vi "HeatFlow HW Conf Save.vi"(8 "HeatFlow HW Cfg":T1, 10 "Conf File":path) -> (0 "error out":errorcluster)   [LabVIEW 2019, in "Acquisition.lvlib"]
uses:
  Acquisition.lvlib
  HeatFlow HW Cfg.ctl
  HeatFlow Acq States.ctl
  <vilib>/Utility/config.llb/Write Key (Boolean).vi
  <vilib>/Utility/config.llb/Write Key (Double).vi
  <vilib>/Utility/config.llb/Write Key (String).vi
  <vilib>/Utility/config.llb/NI_LVConfig.lvlib
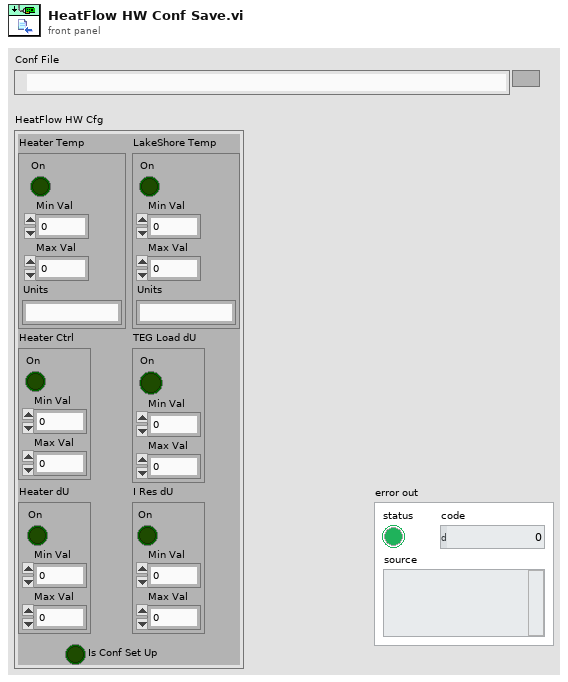
[diagram p1: front panel]
types:
  T1 = typedef "Acquisition.lvlib/HeatFlow HW Cfg.ctl" = cluster{"Heater Temp":cluster{"On":bool, "Min Val":dbl, "Max Val":dbl, "Units":string}, "LakeShore Temp":cluster{"On":bool, "Min Val":dbl, "Max Val":dbl, "Units":string}, "Heater Ctrl":cluster{"On":bool, "Min Val":dbl, "Max Val":dbl}, "TEG Load dU":cluster{"On":bool, "Min Val":dbl, "Max Val":dbl}, "Heater dU":cluster{"On":bool, "Min Val":dbl, "Max Val":dbl}, "I Res dU":cluster{"On":bool, "Min Val":dbl, "Max Val":dbl}, "Is Conf Set Up":bool}
  T2 = typedef "Acquisition.lvlib/HeatFlow Acq States.ctl" = enum16{"Start", "--- Control ---", "HeaterTemp", "DoControl?", "HeaterCtrl", "--- Readings ---", "DoReadings?", "I_Res_dU", "LakeShoreTemp", "Heater_dU", "TEG_Load_dU", "Calculations", "End"}
  T3 = typedef "NI_LVConfig.lvlib/Config Data RefNum.ctl" = refnum<k1>
  T4 = cluster{"On":bool, "Min Val":dbl, "Max Val":dbl, "Units":string}
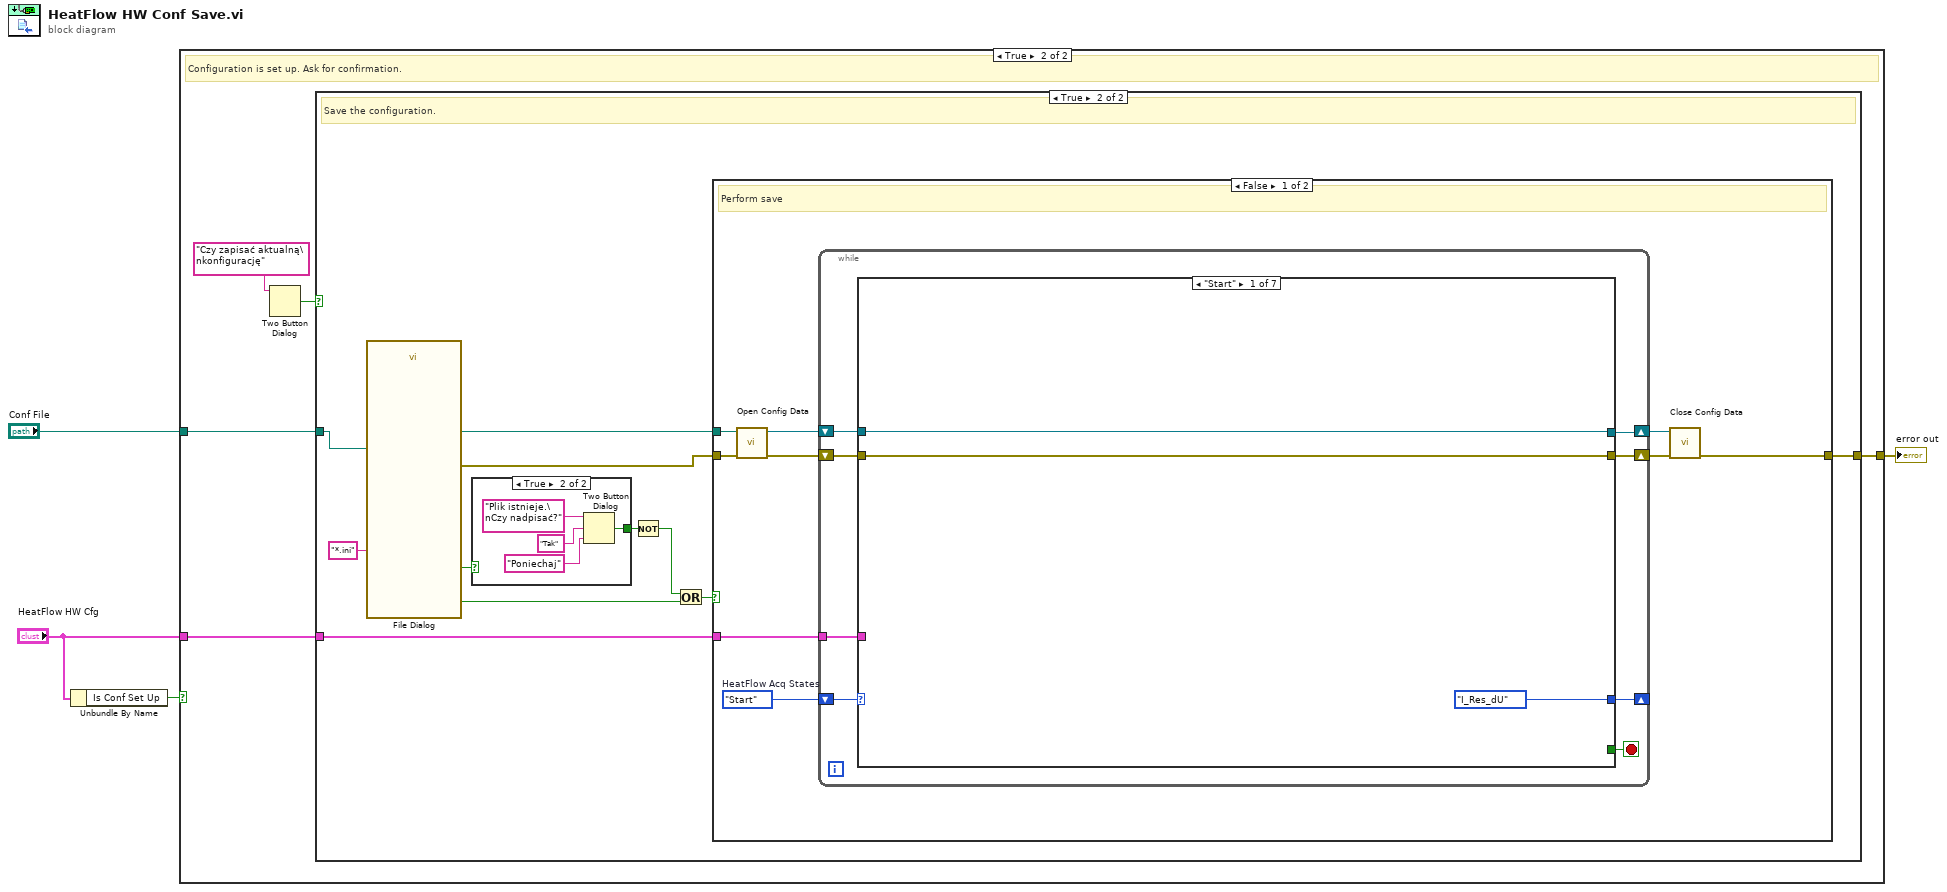
[diagram p0: block diagram]
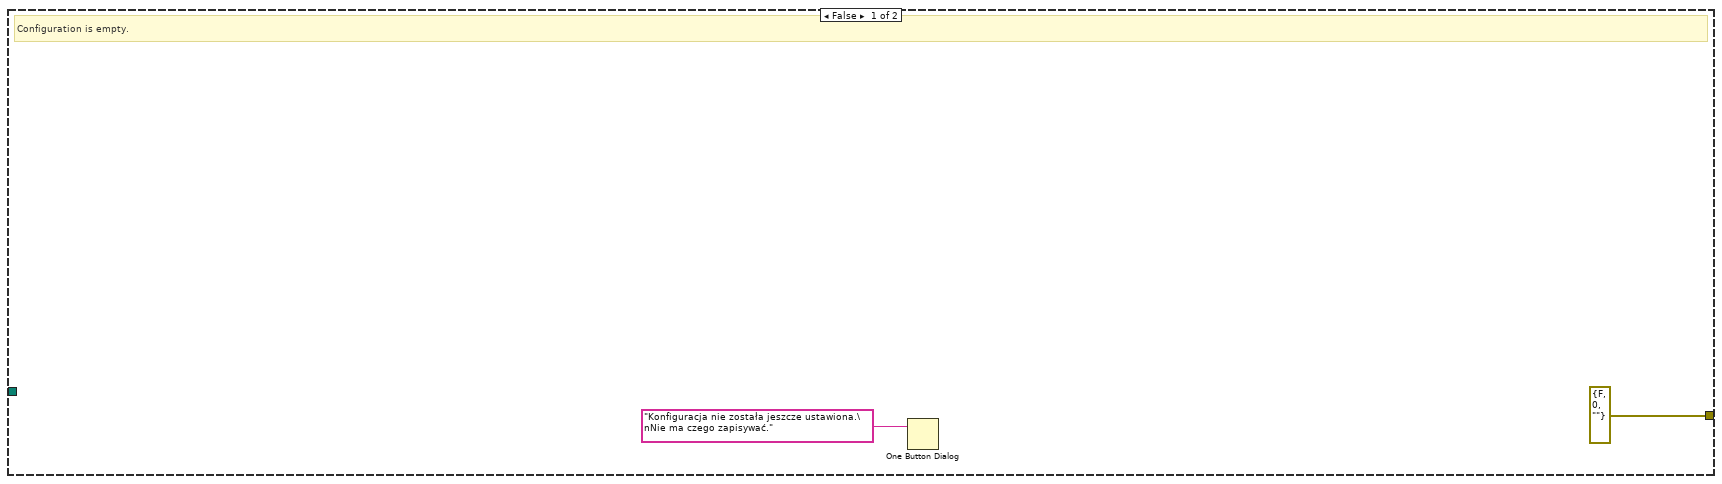
[diagram p2: hidden frame]
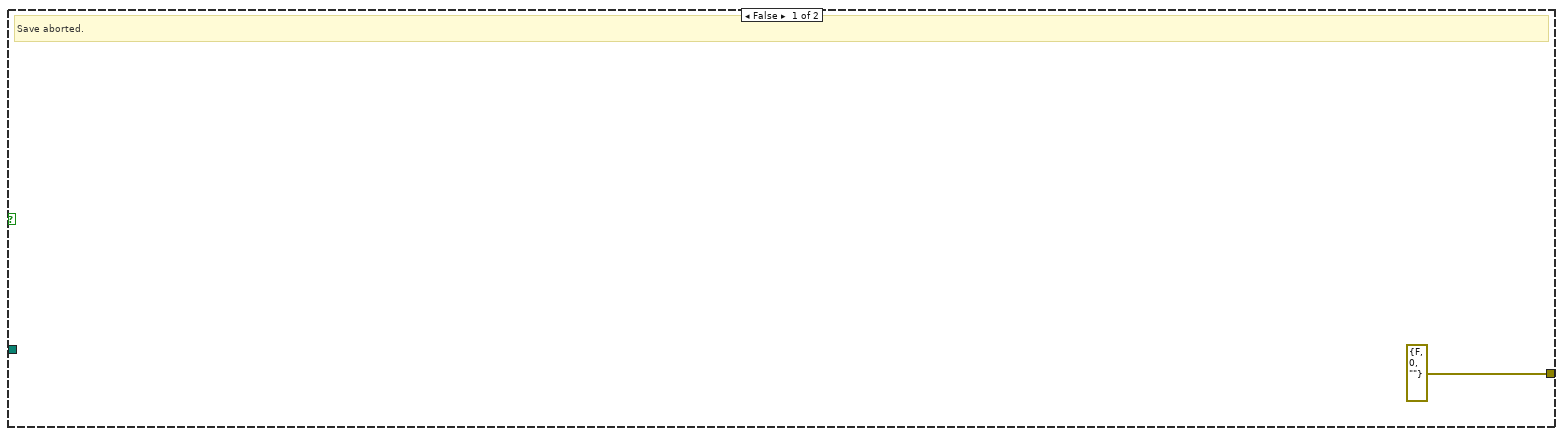
[diagram p3: hidden frame]
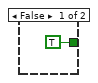
[diagram p4: hidden frame]
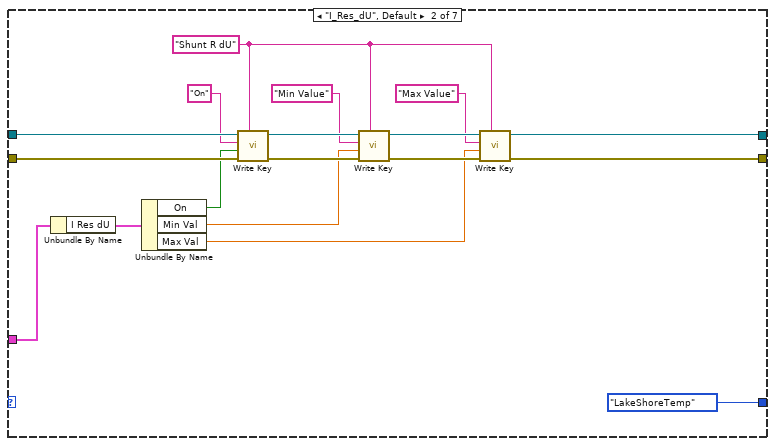
[diagram p5: hidden frame]
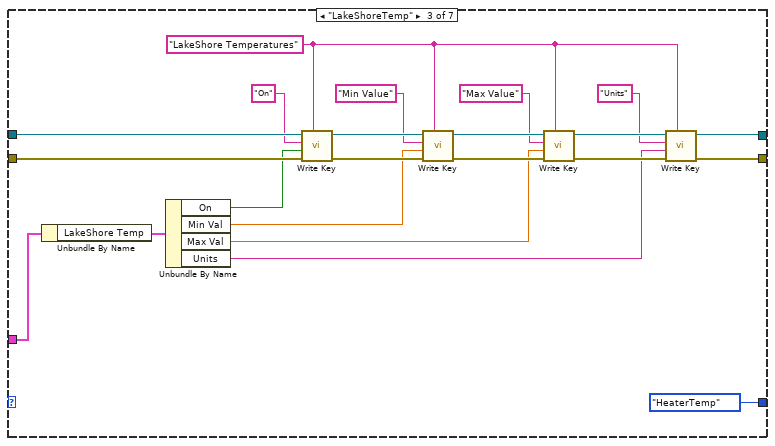
[diagram p6: hidden frame]
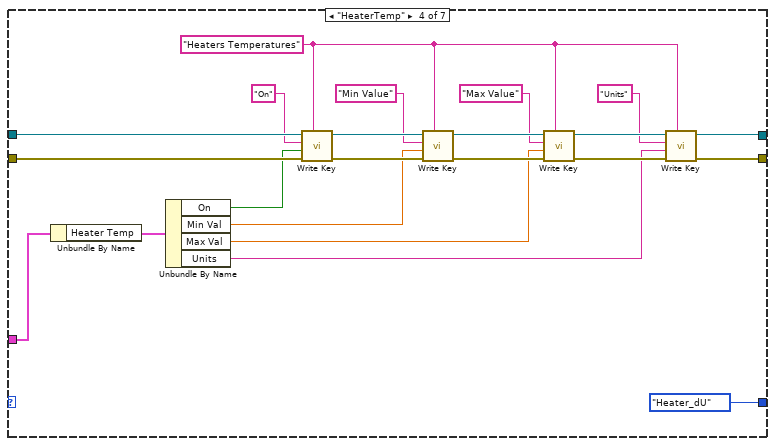
[diagram p7: hidden frame]
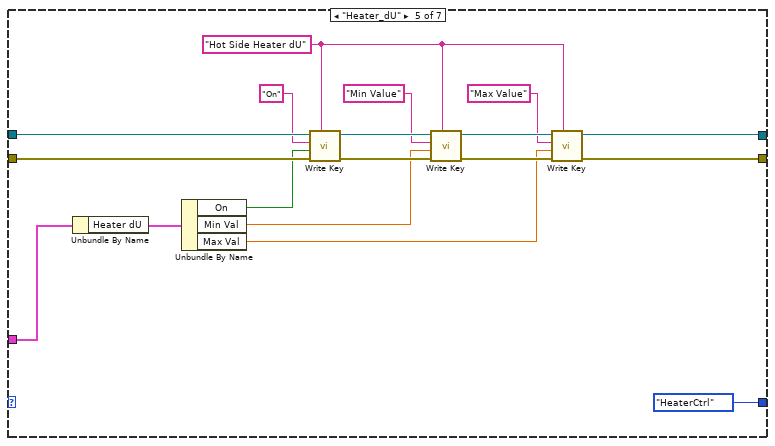
[diagram p8: hidden frame]
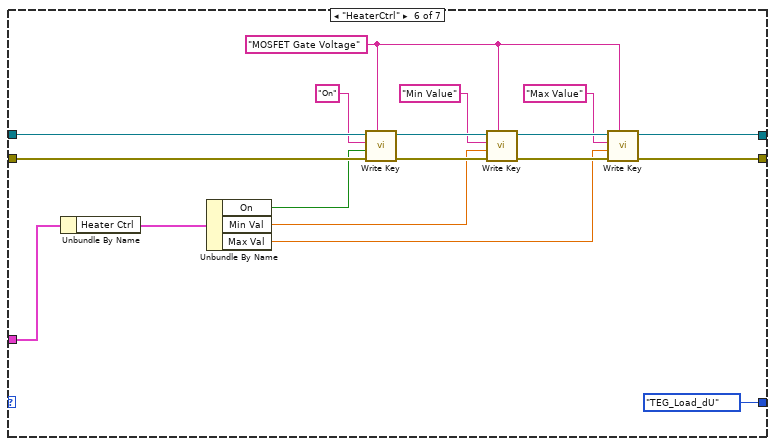
[diagram p9: hidden frame]
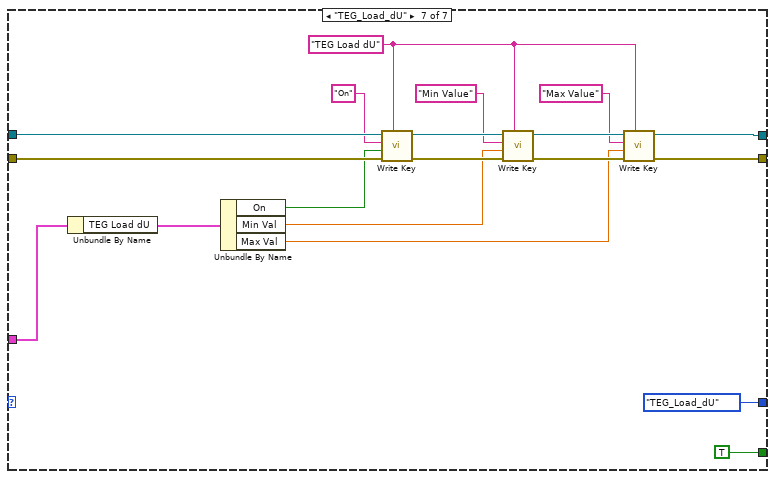
[diagram p10: hidden frame]
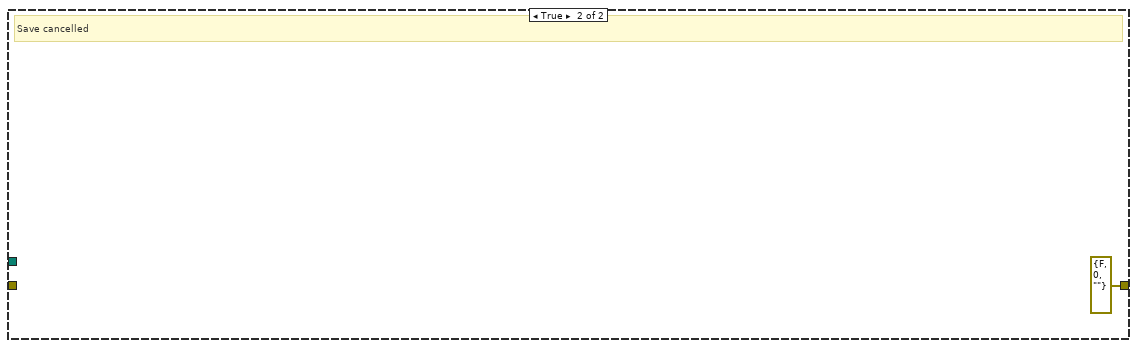
[diagram p11: hidden frame]
diagram:
  n1 = Unbundle By Name("HeatFlow HW Cfg") -> ("Is Conf Set Up"=w2:bool)
  n2 = case shown="True" w2 {
    tunnel: [errorcluster {"status"=FALSE, "code"=0, "source"=""} ("error out") w11] -> w4
    tunnel: "Conf File" -> [_ w10]
    tunnel: "HeatFlow HW Cfg" -> [_ w9]
    frame False {
      # "Configuration is empty."
      n3 = One Button Dialog(message="Konfiguracja nie została jeszcze ustawiona.\nNie ma czego zapisywać.") -> ()  [unwired: 1 in, 1 out]
    }
    frame True {
      # "Configuration is set up. Ask for confirmation."
      n4 = Two Button Dialog(message="Czy zapisać aktualną\nkonfigurację") -> (T button?=w8:bool)  [unwired: 2 in]
      n5 = case shown="True" w8 {
        tunnel: [errorcluster {"status"=FALSE, "code"=0, "source"=""} ("error out") w23] -> w11
        tunnel: w10 -> [_ w20]
        tunnel: w9 -> [_ w22]
        frame False {
          # "Save aborted."
        }
        frame True {
          # "Save the configuration."
          n6 = call "File Dialog"("start path"=w20, "pattern (all files)"="*.ini") -> ("selected path"=w21:path, "exists"=w17:bool, "cancelled"=w13:bool, "error out"=w19:errorcluster)  [unwired: 10 in]
          n7 = case shown="True" w17 {
            tunnel: [TRUE ("T button?") w25] -> w16
            frame False {
            }
            frame True {
              n8 = Two Button Dialog(message="Plik istnieje.\nCzy nadpisać?", 1:"Poniechaj" ("F button name (\"Cancel\")"), 2:"Tak" ("T button name (\"OK\")")) -> (T button?=w25:bool)
            }
          }
          n9 = Not(x=w16) -> (.not. x?=w14:bool)
          n10 = Or(x=w14, y=w13) -> (x .or. y?=w15:bool)
          n11 = case shown="False" w15 {
            tunnel: [w32 errorcluster {"status"=FALSE, "code"=0, "source"=""} ("error out")] -> w23
            tunnel: w22 -> [w31 _]
            tunnel: w21 -> [w30 _]
            tunnel: w19 -> [w29 _]
            frame False {
              w37 = HeatFlow_Acq_States."Start"  # HeatFlow Acq States
              # "Perform save"
              n12 = call <vilib>:"Open Config Data.vi"("error in (no error)"=w29, "configuration file path"=w30) -> ("error out"=w35:errorcluster, "refnum"=w36:T3)  [unwired: 7 in, 1 out]
              n13 = while {
                shift-right: [w44] -> _
                shift-left: w37 -> [w45]
                shift-right: [w40] -> w34
                shift-left: w35 -> [w41]
                shift-right: [w39] -> w33
                shift-left: w36 -> [w43]
                tunnel: w31 -> [w42]
                stop <- w38 stop-if-true
                n14 = case shown="\"Start\"" w45 {
                  tunnel: [HeatFlow_Acq_States."I_Res_dU" ("Measurement States") HeatFlow_Acq_States."LakeShoreTemp" ("Measurement States") HeatFlow_Acq_States."HeaterTemp" ("Measurement States") HeatFlow_Acq_States."Heater_dU" ("Measurement States") HeatFlow_Acq_States."HeaterCtrl" ("Measurement States") HeatFlow_Acq_States."TEG_Load_dU" ("Measurement States") HeatFlow_Acq_States."TEG_Load_dU" ("Measurement States")] -> w44
                  tunnel: w43 -> [w47 w65 w87 w109 w127 w145 w164]
                  tunnel: w42 -> [_ w55 w72 w94 w117 w135 w154]
                  tunnel: w41 -> [w46 w64 w86 w108 w126 w144 w163]
                  tunnel: [w46 w50 w78 w100 w112 w130 w149] -> w40
                  tunnel: [w47 w51 w82 w104 w113 w131 w150] -> w39
                  tunnel: [_ _ _ _ _ _ TRUE] -> w38
                  frame "Start" {
                  }
                  frame "I_Res_dU", Default {
                    w59 = "Shunt R dU" ("section")
                    n15 = Unbundle By Name(w55) -> ("I Res dU"=w49:cluster{"On":bool, "Min Val":dbl, "Max Val":dbl})
                    n16 = Unbundle By Name(w49) -> ("On"=w54:bool, "Min Val"=w53:dbl, "Max Val"=w52:dbl)
                    n17 = call-poly <vilib>:"Write Key.vi"("section"=w59, "error in (no error)"=w64, "value"=w54, "key"="On", "refnum"=w65) -> ("error out"=w61:errorcluster, "refnum out"=w63:T3)  [unwired: 4 in, 1 out]
                    n18 = call-poly <vilib>:"Write Key.vi"("section"=w59, "error in (no error)"=w61, "value"=w53, "key"="Min Value", "refnum"=w63) -> ("error out"=w60:errorcluster, "refnum out"=w62:T3)  [unwired: 4 in, 1 out]
                    n19 = call-poly <vilib>:"Write Key.vi"("section"=w59, "error in (no error)"=w60, "value"=w52, "key"="Max Value", "refnum"=w62) -> ("error out"=w50:errorcluster, "refnum out"=w51:T3)  [unwired: 4 in, 1 out]
                  }
                  frame "LakeShoreTemp" {
                    w77 = "LakeShore Temperatures" ("section")
                    n20 = Unbundle By Name(w72) -> ("LakeShore Temp"=w67:T4)
                    n21 = Unbundle By Name(w67) -> ("On"=w71:bool, "Min Val"=w70:dbl, "Max Val"=w69:dbl, "Units"=w68:string)
                    n22 = call-poly <vilib>:"Write Key.vi"("section"=w77, "error in (no error)"=w86, "value"=w71, "key"="On", "refnum"=w87) -> ("error out"=w81:errorcluster, "refnum out"=w85:T3)  [unwired: 4 in, 1 out]
                    n23 = call-poly <vilib>:"Write Key.vi"("section"=w77, "error in (no error)"=w81, "value"=w70, "key"="Min Value", "refnum"=w85) -> ("error out"=w80:errorcluster, "refnum out"=w84:T3)  [unwired: 4 in, 1 out]
                    n24 = call-poly <vilib>:"Write Key.vi"("section"=w77, "error in (no error)"=w80, "value"=w69, "key"="Max Value", "refnum"=w84) -> ("error out"=w79:errorcluster, "refnum out"=w83:T3)  [unwired: 4 in, 1 out]
                    n25 = call-poly <vilib>:"Write Key.vi"("section"=w77, "error in (no error)"=w79, "value"=w68, "key"="Units", "refnum"=w83) -> ("error out"=w78:errorcluster, "refnum out"=w82:T3)  [unwired: 4 in, 1 out]
                  }
                  frame "HeaterTemp" {
                    w99 = "Heaters Temperatures" ("section")
                    n26 = Unbundle By Name(w94) -> ("Heater Temp"=w89:T4)
                    n27 = Unbundle By Name(w89) -> ("On"=w93:bool, "Min Val"=w92:dbl, "Max Val"=w91:dbl, "Units"=w90:string)
                    n28 = call-poly <vilib>:"Write Key.vi"("section"=w99, "error in (no error)"=w108, "value"=w93, "key"="On", "refnum"=w109) -> ("error out"=w103:errorcluster, "refnum out"=w107:T3)  [unwired: 4 in, 1 out]
                    n29 = call-poly <vilib>:"Write Key.vi"("section"=w99, "error in (no error)"=w103, "value"=w92, "key"="Min Value", "refnum"=w107) -> ("error out"=w102:errorcluster, "refnum out"=w106:T3)  [unwired: 4 in, 1 out]
                    n30 = call-poly <vilib>:"Write Key.vi"("section"=w99, "error in (no error)"=w102, "value"=w91, "key"="Max Value", "refnum"=w106) -> ("error out"=w101:errorcluster, "refnum out"=w105:T3)  [unwired: 4 in, 1 out]
                    n31 = call-poly <vilib>:"Write Key.vi"("section"=w99, "error in (no error)"=w101, "value"=w90, "key"="Units", "refnum"=w105) -> ("error out"=w100:errorcluster, "refnum out"=w104:T3)  [unwired: 4 in, 1 out]
                  }
                  frame "Heater_dU" {
                    w121 = "Hot Side Heater dU" ("section")
                    n32 = Unbundle By Name(w117) -> ("Heater dU"=w111:cluster{"On":bool, "Min Val":dbl, "Max Val":dbl})
                    n33 = Unbundle By Name(w111) -> ("On"=w116:bool, "Min Val"=w115:dbl, "Max Val"=w114:dbl)
                    n34 = call-poly <vilib>:"Write Key.vi"("section"=w121, "error in (no error)"=w126, "value"=w116, "key"="On", "refnum"=w127) -> ("error out"=w123:errorcluster, "refnum out"=w125:T3)  [unwired: 4 in, 1 out]
                    n35 = call-poly <vilib>:"Write Key.vi"("section"=w121, "error in (no error)"=w123, "value"=w115, "key"="Min Value", "refnum"=w125) -> ("error out"=w122:errorcluster, "refnum out"=w124:T3)  [unwired: 4 in, 1 out]
                    n36 = call-poly <vilib>:"Write Key.vi"("section"=w121, "error in (no error)"=w122, "value"=w114, "key"="Max Value", "refnum"=w124) -> ("error out"=w112:errorcluster, "refnum out"=w113:T3)  [unwired: 4 in, 1 out]
                  }
                  frame "HeaterCtrl" {
                    w139 = "MOSFET Gate Voltage" ("section")
                    n37 = Unbundle By Name(w135) -> ("Heater Ctrl"=w129:cluster{"On":bool, "Min Val":dbl, "Max Val":dbl})
                    n38 = Unbundle By Name(w129) -> ("On"=w134:bool, "Min Val"=w133:dbl, "Max Val"=w132:dbl)
                    n39 = call-poly <vilib>:"Write Key.vi"("section"=w139, "error in (no error)"=w144, "value"=w134, "key"="On", "refnum"=w145) -> ("error out"=w141:errorcluster, "refnum out"=w143:T3)  [unwired: 4 in, 1 out]
                    n40 = call-poly <vilib>:"Write Key.vi"("section"=w139, "error in (no error)"=w141, "value"=w133, "key"="Min Value", "refnum"=w143) -> ("error out"=w140:errorcluster, "refnum out"=w142:T3)  [unwired: 4 in, 1 out]
                    n41 = call-poly <vilib>:"Write Key.vi"("section"=w139, "error in (no error)"=w140, "value"=w132, "key"="Max Value", "refnum"=w142) -> ("error out"=w130:errorcluster, "refnum out"=w131:T3)  [unwired: 4 in, 1 out]
                  }
                  frame "TEG_Load_dU" {
                    w158 = "TEG Load dU" ("section")
                    n42 = Unbundle By Name(w154) -> ("TEG Load dU"=w147:cluster{"On":bool, "Min Val":dbl, "Max Val":dbl})
                    n43 = Unbundle By Name(w147) -> ("On"=w153:bool, "Min Val"=w152:dbl, "Max Val"=w151:dbl)
                    n44 = call-poly <vilib>:"Write Key.vi"("section"=w158, "error in (no error)"=w163, "value"=w153, "key"="On", "refnum"=w164) -> ("error out"=w160:errorcluster, "refnum out"=w162:T3)  [unwired: 4 in, 1 out]
                    n45 = call-poly <vilib>:"Write Key.vi"("section"=w158, "error in (no error)"=w160, "value"=w152, "key"="Min Value", "refnum"=w162) -> ("error out"=w159:errorcluster, "refnum out"=w161:T3)  [unwired: 4 in, 1 out]
                    n46 = call-poly <vilib>:"Write Key.vi"("section"=w158, "error in (no error)"=w159, "value"=w151, "key"="Max Value", "refnum"=w161) -> ("error out"=w149:errorcluster, "refnum out"=w150:T3)  [unwired: 4 in, 1 out]
                  }
                }
              }
              n47 = call <vilib>:"Close Config Data.vi"("error in (no error)"=w34, "refnum"=w33) -> ("error out"=w32:errorcluster)  [unwired: 8 in, 1 out]
            }
            frame True {
              # "Save cancelled"
            }
          }
        }
      }
    }
  }
  "error out" <- w4
